vi "Measurement Conversion.vi"(6 "Conversion into microns":dbl, 7 "Pixel Measurement at Calibration":dbl format="%#_13g", 8 "Left Spindle Pixel measurement from OUI":dbl, 9 "Centre Spindle Pixel measurement from OUI":dbl, 10 "Right Spindle Pixel measurement from OUI":dbl, 11 "Dimension of Standard in mm":dbl format="%#_13g") -> (0 "Left Spindle Measurement in microns":dbl, 1 "Center Spindle Measurement in microns":dbl, 2 "Right Measurement in microns":dbl, 3 "Pixel Size Coefficient":dbl)   [LabVIEW 2016]
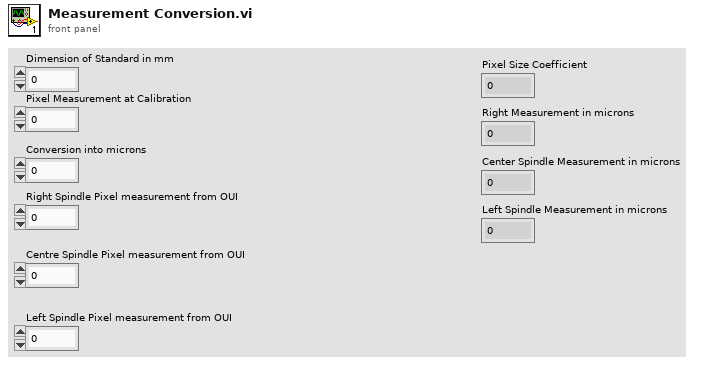
[diagram p1: front panel]
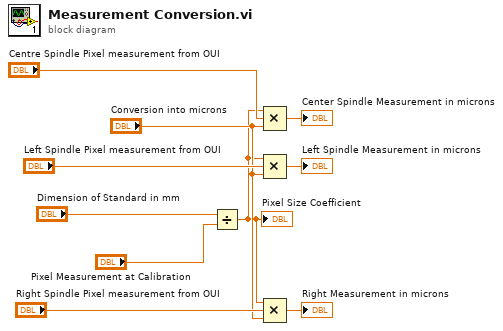
[diagram p0: block diagram]
diagram:
  n1 = Divide(x="Dimension of Standard in mm", y="Pixel Measurement at Calibration") -> (x/y=w1:dbl)
  "Pixel Size Coefficient" <- w1
  n2 = Compound Arithmetic op=MULTIPLY(w1, "Centre Spindle Pixel measurement from OUI", "Conversion into microns") -> (→"Center Spindle Measurement in microns":dbl)
  n3 = Compound Arithmetic op=MULTIPLY(w1, "Left Spindle Pixel measurement from OUI", "Conversion into microns") -> (→"Left Spindle Measurement in microns":dbl)
  n4 = Compound Arithmetic op=MULTIPLY(w1, "Right Spindle Pixel measurement from OUI", "Conversion into microns") -> (→"Right Measurement in microns":dbl)
